vi "histogram_v23-malusBook.vi"(6 "ROI Descriptor":T2 {"Contours"."Type" items=["No Selection", "Point", "Line", "Rectangle", "Oval", "Polygon", "Freehand Region", "Annulus", "Unused2", "Unused3", "Broken Line", "Freehand Line", "Rotated Rectangle"]}, 8 "useROI":bool, 9 "Color":bool, 10 "14bits":bool, 11 "Image":T1) -> (0 "error out":errorcluster, 1 "# Sat. Pixels":sgl(slide) scale=0.0..10.0, 2 "mean (ROI)":dbl, 3 "Histograph":T3(graph)={"Starting Value"=-32768.0, "Incremental Value"=1.0, "Histogram"=array[65536 elements]}, 4 "image_size":i32, 5 "max (ROI)":i16, 7 "max_counts":dbl)   [LabVIEW 2022 SP3]
uses:
  <vilib>/vision/Image Controls.llb/IMAQ Image.ctl
  <vilib>/vision/NI_Vision_Development_Module.lvlib
panel:
  out "Image Out":T1
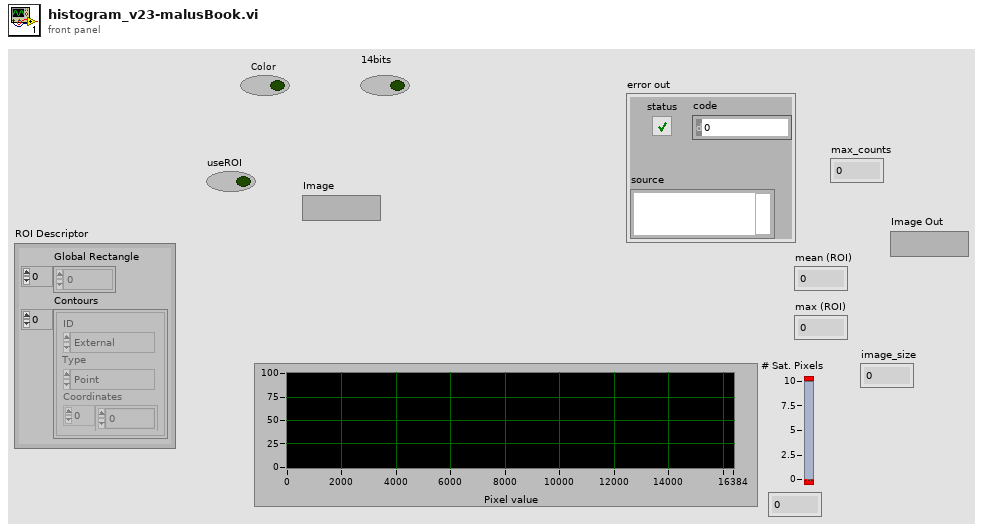
[diagram p1: front panel]
types:
  T1 = typedef "IMAQ Image.ctl" = refnum<image>
  T2 = cluster{"Global Rectangle":i32[], "Contours":cluster{"ID":enum32{"External", "Internal"}, "Type":u32, "Coordinates":i32[]}[]}
  T3 = cluster{"Starting Value":sgl, "Incremental Value":sgl, "Histogram":u32[]}
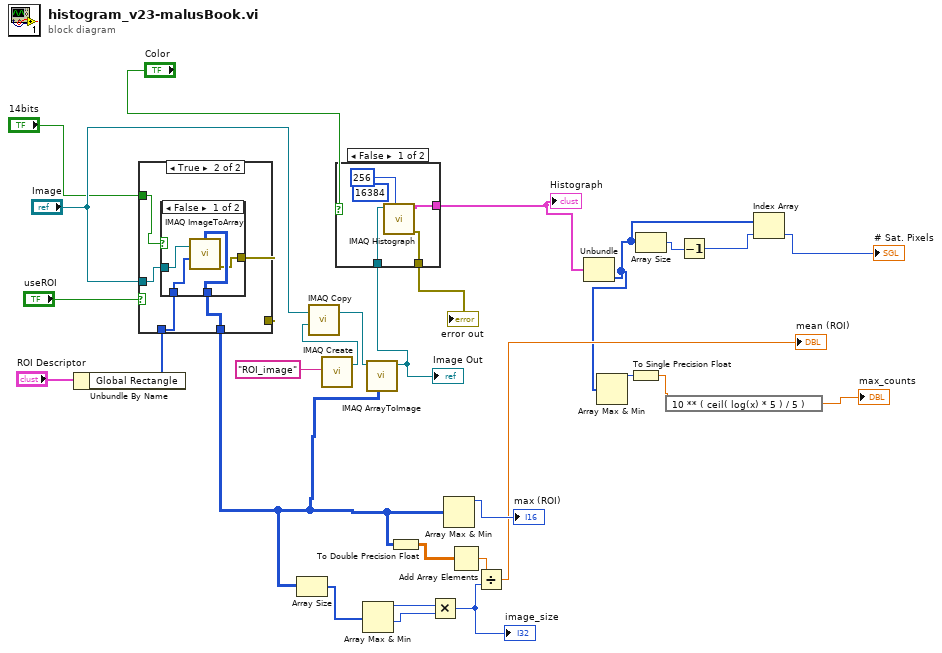
[diagram p0: block diagram]
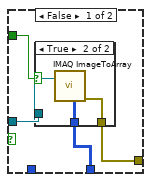
[diagram p2: hidden frame]
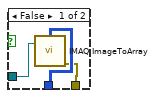
[diagram p3: hidden frame]
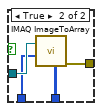
[diagram p4: hidden frame]
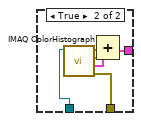
[diagram p5: hidden frame]
diagram:
  n1 = Unbundle By Name("ROI Descriptor") -> ("Global Rectangle"=w22:i32[])
  n2 = case shown="True" "useROI" {
    tunnel: [w32 w41] -> w10
    tunnel: w22 -> [_ w42]
    tunnel: "Image" -> [w30 w43]
    tunnel: [w31 w40] -> _
    tunnel: "14bits" -> [w29 w39]
    frame False {
      n3 = case shown="True" w29 {
        tunnel: [w35 w38] -> w32
        tunnel: [w33 w37] -> w31
        tunnel: w30 -> [w34 w36]
        frame False {
          n4 = call "IMAQ ImageToArray"("Image"=w34) -> ("error out"=w33:errorcluster, "Image Pixels (U8)"=w35:u8[][])  [unwired: 3 in, 3 out]
        }
        frame True {
          n5 = call "IMAQ ImageToArray"("Image"=w36) -> ("Image Pixels (U16)"=w38:u16[][], "error out"=w37:errorcluster)  [unwired: 3 in, 3 out]
        }
      }
    }
    frame True {
      n6 = case shown="False" w39 {
        tunnel: w43 -> [w47 w51]
        tunnel: w42 -> [w44 w50]
        tunnel: [w46 w49] -> w41
        tunnel: [w45 w48] -> w40
        frame False {
          n7 = call "IMAQ ImageToArray"("Optional Rectangle"=w44, "Image"=w47) -> ("error out"=w45:errorcluster, "Image Pixels (U8)"=w46:u8[][])  [unwired: 2 in, 3 out]
        }
        frame True {
          n8 = call "IMAQ ImageToArray"("Optional Rectangle"=w50, "Image"=w51) -> ("Image Pixels (U16)"=w49:u16[][], "error out"=w48:errorcluster)  [unwired: 2 in, 3 out]
        }
      }
    }
  }
  n9 = Array Size(array=w10) -> (size(s)=w16:i32[])
  n10 = call "IMAQ Create"("Image Name"="ROI_image") -> ("New Image"=w7:T1)  [unwired: 4 in, 1 out]
  n11 = call "IMAQ Copy"("Image Dst"=w7, "Image Src"="Image") -> ("Image Dst Out"=w6:T1)  [unwired: 4 in, 1 out]
  n12 = Array Max & Min(array=w16) -> (max value=w15:i32, min value=w11:i32)  [unwired: 2 out]
  n13 = call "IMAQ ArrayToImage"("Image Pixels (U16)"=w10, "Image"=w6) -> ("Image Out"=w9:T1)  [unwired: 8 in, 1 out]
  "Image Out" <- w9
  n14 = case shown="False" "Color" {
    tunnel: [w55 w58] -> w27
    tunnel: [w54 w57] -> w25
    tunnel: w9 -> [w53 w56]
    frame False {
      (unwired) 16384 ("Number of Classes")
      n15 = call "IMAQ Histograph"("Number of Classes"=256, "Image"=w53) -> ("error out"=w54:errorcluster, "Histogram Graph"=w55:T3)  [unwired: 6 in, 2 out]
    }
    frame True {
      n16 = call "IMAQ ColorHistograph"("Image Src"=w56) -> ("Red or Hue Histogram Graph"=w61:T3, "Green or Sat Histogram Graph"=w60:T3, "Blue or Luma or Val or Inten Histogram Graph"=w59:T3, "error out"=w57:errorcluster)  [unwired: 5 in]
      n17 = Compound Arithmetic op=ADD(w61, w60, w59) -> (w58:T3)
    }
  }
  "Histograph" <- w27
  "error out" <- w25
  n18 = To Double Precision Float(number=w10) -> (double precision float=w12:dbl[][])
  n19 = Multiply(x=w15, y=w11) -> (x*y=w14:i32)
  "image_size" <- w14
  n20 = Array Max & Min(array=w10) -> (max value=→"max (ROI)":u16)  [unwired: 3 out]
  n21 = Add Array Elements(numeric array=w12) -> (sum=w17:dbl)
  n22 = Divide(x=w17, y=w14) -> (x/y=→"mean (ROI)":dbl)
  n23 = Unbundle(w27) -> ("Histogram"=w5:u32[])  [unwired: 2 out]
  n24 = Array Max & Min(array=w5) -> (max value=w4:u32)  [unwired: 3 out]
  n25 = To Single Precision Float(number=w4) -> (single precision float=w3:sgl)
  n26 = Array Size(array=w5) -> (size(s)=w23:i32)
  n27 = expression code="10 ** ( ceil( log(x) * 5 ) / 5 )"(w3) -> (→"max_counts":sgl)
  n28 = Decrement(x=w23) -> (x-1=w24:i32)
  n29 = Index Array(array=w5, index=w24) -> (element=→"# Sat. Pixels":u32)
